vi "Enqueue ActorRef.vi"(8 "error in (no error)":errorcluster, 9 "UIRef":refnum<class "Message Enqueuer.lvclass">, 11 "MainUI in":refnum<class "MainUI.lvclass">) -> (0 "error out":errorcluster, 3 "MainUI out":refnum<class "MainUI.lvclass">)   [LabVIEW 2019, in "MainUI.lvlib" / "MainUI.lvclass"]
uses:
  MainUI.lvclass
  <vilib>/ActorFramework/Message Enqueuer/Message Enqueuer.lvclass
  ModuleAbstract/ModuleAbstract.lvclass
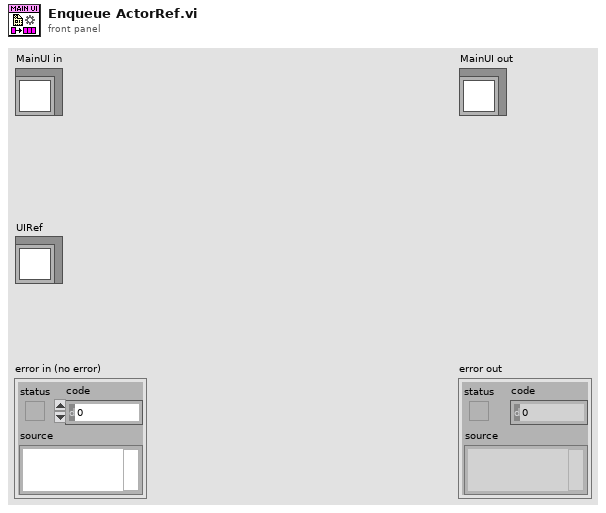
[diagram p1: front panel]
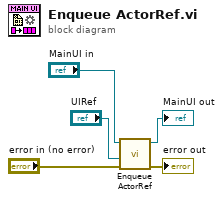
[diagram p0: block diagram]
diagram:
  n1 = call-parent "Enqueue ActorRef.vi"("error in (no error)"="error in (no error)", "UIRef"="UIRef", "ModuleAbstract in"="MainUI in") -> ("error out"=→"error out":errorcluster, "ModuleAbstract out"=→"MainUI out":refnum<class "MainUI.lvclass">)  [unwired: 7 in]
